vi "ReadCom1.vi"(8 "error in (no error)":errorcluster, 11 "Data In":T3) -> (0 "error out":errorcluster, 1 "Next State":T2=enum."State1", 2 "States":T1, 3 "Data Out":T3)   [LabVIEW 2013]
uses:
  controls/Data.ctl
  controls/Wait Scan States.ctl
  controls/State.ctl
panel:
  # "日期"
  # "機種名稱"
  # "機種代號"
  # "商品條碼"
  # "OK"
  # "台"
  # "NG"
  # "總計"
  # "台"
  # "日期"
  # "機種名稱"
  # "機種代號"
  # "商品條碼"
  # "OK"
  # "台"
  # "NG"
  # "總計"
  # "台"
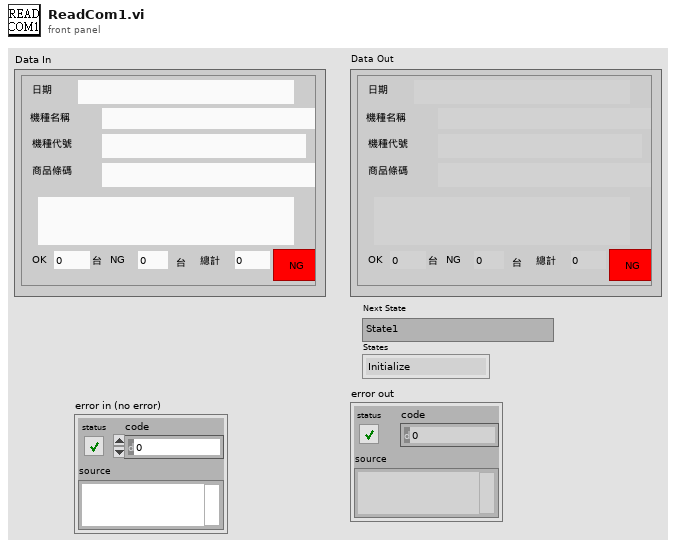
[diagram p1: front panel]
types:
  T1 = typedef "State.ctl" = enum16{"Initialize", "Wait for Scan", "State 1", "State 2", "OKNG", "Exit"}
  T2 = typedef "Wait Scan States.ctl" = enum16{"Initialize", "State1", "Stop"}
  T3 = typedef "Data.ctl" = cluster{"Date":string, "BarCode1":string, "BarCode2":string, "BarCode3":string, "Message":string, "OK Count":u16, "NG Count":u16, "Total Count":u16, "ModelData":string[][], "OK&NG":bool, "COM1":refnum<visa-resource-name>, "COM2":refnum<visa-resource-name>, "IO":i32}
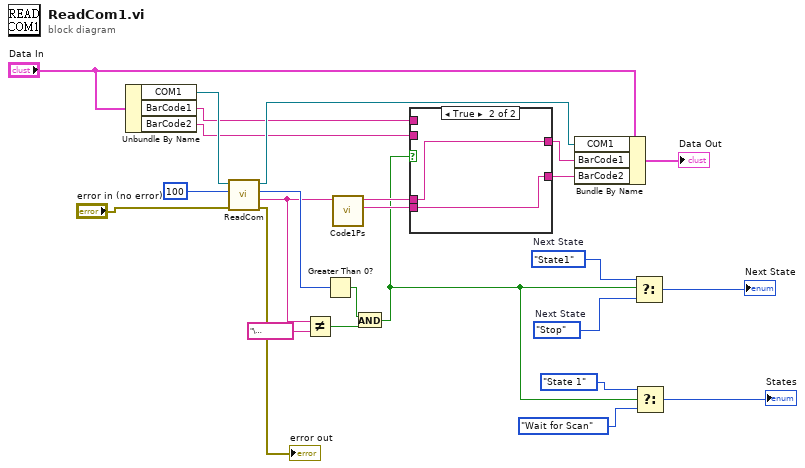
[diagram p0: block diagram]
diagram:
  w21 = Wait_Scan_States."State1"  # Next State
  w20 = Wait_Scan_States."Stop"  # Next State
  n1 = Unbundle By Name("Data In") -> ("COM1"=w25:refnum<visa-resource-name>, "BarCode1"=w9:string, "BarCode2"=w8:string)
  n2 = call "ReadCom.vi"("error in (no error)"="error in (no error)", "delay before read (ms)"=u32 100, "Com In"=w25) -> ("error out"=→"error out":errorcluster, "Response"=w3:string, "bytes read"=w19:u32, "Com Out"=w12:refnum<visa-resource-name>)  [unwired: 5 in]
  n3 = Not Equal?(x=w3, y="\u0002NoRead\u0003") -> (x != y?=w1:bool)
  n4 = Greater Than 0?(x=w19) -> (x > 0?=w5:bool)
  n5 = call "Code1Ps.vi"("Code1 In"=w3) -> ("機種代號"=w10:string, "機種名"=w11:string)  [unwired: 8 in, 1 out]
  n6 = And(x=w5, y=w1) -> (x .and. y?=w4:bool)
  n7 = case shown="True" w4 {
    tunnel: w11 -> [_ w29]
    tunnel: w10 -> [_ w28]
    tunnel: w9 -> [w27 _]
    tunnel: w8 -> [w26 _]
    tunnel: [w27 w29] -> w7
    tunnel: [w26 w28] -> w6
    frame False {
    }
    frame True {
    }
  }
  n8 = Bundle By Name(cluster="Data In", "COM1"=w12, "BarCode1"=w7, "BarCode2"=w6) -> (→"Data Out":T3)
  n9 = Select(t=w21, s=w4, f=w20) -> (s? t:f=→"Next State":T2)
  n10 = Select(t=State."State 1" ("States"), s=w4, f=State."Wait for Scan" ("States")) -> (s? t:f=→"States":T1)
